vi "Open NameParameter.vi"(11 "Parameter Path":path) -> (0 "NamePara Out":string[](array[string]), 2 "File OK":bool, 3 "dup path":path)   [LabVIEW 2017]
uses:
  <vilib>/Utility/file.llb/Read Delimited Spreadsheet (string).vi
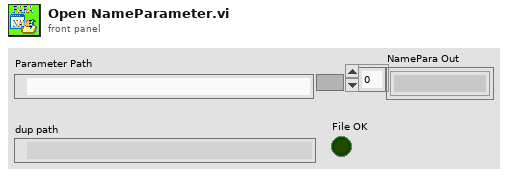
[diagram p1: front panel]
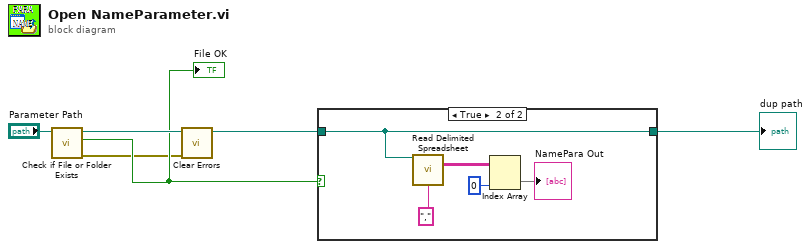
[diagram p0: block diagram]
diagram:
  n1 = call <vilib>:"Check if File or Folder Exists.vi"("path"="Parameter Path") -> ("error out"=w2:errorcluster, "file or folder exists?"=w4:bool, "dup path"=w5:path)  [unwired: 8 in]
  "File OK" <- w4
  n2 = call <vilib>:"Clear Errors.vi"("error in (no error)"=w2) -> ()  [unwired: 5 in, 2 out]
  n3 = case shown="True" w4 {
    tunnel: w5 -> [w6 w8]
    tunnel: [w6 w8] -> w1
    frame False {
    }
    frame True {
      n4 = call-poly <vilib>:"Read Delimited Spreadsheet.vi"("file path (dialog if empty)"=w8, "delimiter (\\t)"="," ("delimiter (\\t)")) -> ("all rows"=w10:string[][])  [unwired: 8 in, 5 out]
      n5 = Index Array(array=w10, index (col)=0 ("disabled index (col)")) -> (element=→"NamePara Out":string[])  [unwired: 1 in]
    }
  }
  "dup path" <- w1
